vi "salto_pag.vi"(11 "reference":refnum<vi>) -> ()   [LabVIEW 2020]
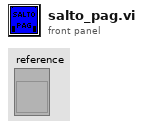
[diagram p1: front panel]
types:
  T1 = enum32{"Bad", "Idle", "Run top level", "Running"}
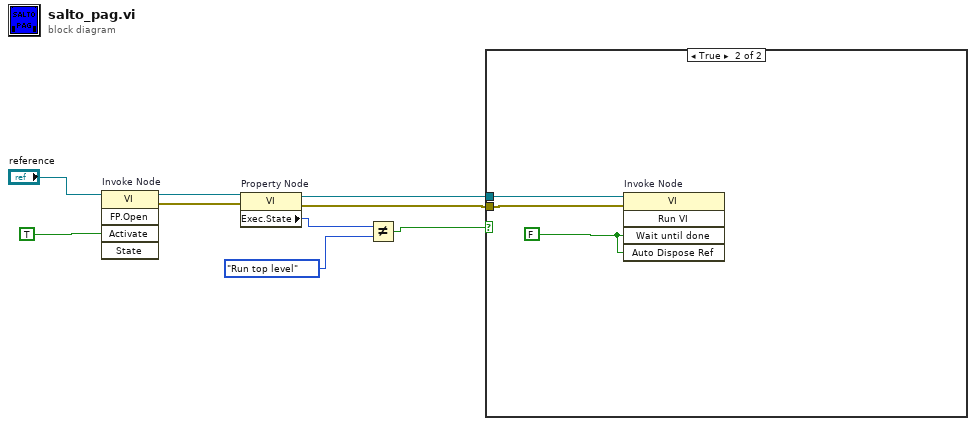
[diagram p0: block diagram]
diagram:
  n1 = invoke on="Invoke Node" class="VI" method="FP.Open"(reference="reference", "Activate"=TRUE ("Activate?")) -> (reference out=w7:refnum<vi>, error out=w6:errorcluster)  [unwired: 3 in, 3 out]
  n2 = property on="Property Node" class="VI"(reference=w7, error in=w6) -> (reference out=w2:refnum<vi>, error out=w1:errorcluster, "Exec.State"=w5:T1)
  n3 = Not Equal?(x=w5, y=T1."Run top level") -> (x != y?=w3:bool)
  n4 = case shown="True" w3 {
    tunnel: w2 -> [_ w12]
    tunnel: w1 -> [_ w11]
    frame False {
    }
    frame True {
      w10 = FALSE ("Wait Until Done")
      n5 = invoke on="Invoke Node" class="VI" method="Run VI"(reference=w12, error in=w11, "Wait until done"=w10, "Auto Dispose Ref"=w10) -> ()  [unwired: 1 in, 5 out]
    }
  }
